vi "test_SomeSessionsRegistered_CallCreateSessionsAndCloseSessionsWithInitializeAndDetach_InitializeAndCloseCalledWithProperBehavior.vi"(11 "error in":errorcluster) -> (4 "pass":bool, 6 "result":string, 15 "error out":errorcluster)   [LabVIEW 2020, in "MeasurementServerTests.lvlib"]
uses:
  MeasurementServerTests.lvlib
  Runtime/MeasurementLink Session Management/Session Reservation/Initialize and Close Session Behavior.ctl
  Runtime/MeasurementLink Session Management/Session Reservation/Session Reservation.lvclass
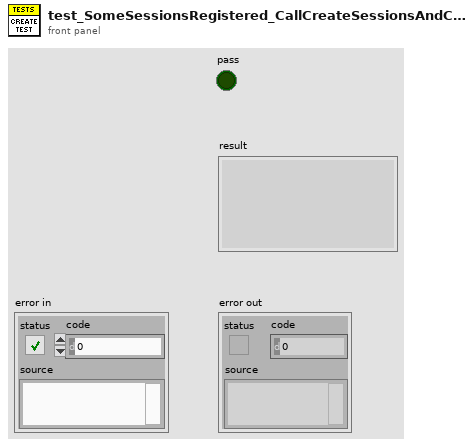
[diagram p1: front panel]
types:
  T1 = typedef "MeasurementLink Session Management.lvlib/Session Reservation.lvclass/Initialize and Close Session Behavior.ctl" = enum16{"Auto", "Initialize and Close", "Attach and Detach", "Initialize and Detach", "Attach and Close"}
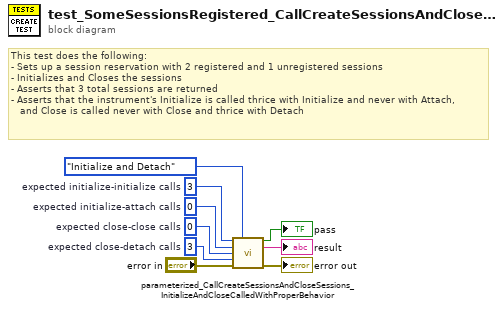
[diagram p0: block diagram]
diagram:
  w5 = u32 3  # expected close-detach calls
  w6 = u32 0  # expected close-close calls
  w7 = u32 0  # expected initialize-attach calls
  w8 = u32 3  # expected initialize-initialize calls
  # "This test does the following:\n- Sets up a session reservation with 2 registered and 1 unregistered sessions\n- Initializes and Closes the sessions\n- Asserts that 3 total sessions are returned\n- Asserts that the instrument's Initialize is called thrice with Initialize and never with Attach,\n   and Close is called never with Close and thrice with Detach"
  n1 = call "parameterized_CallCreateSessionsAndCloseSessions_InitializeAndCloseCalledWithProperBehavior.vi"("expected initialize-initialize calls"=w8, "initialize and close session behavior"=Initialize_and_Close_Session_Behavior."Initialize and Detach", "expected initialize-attach calls"=w7, "expected close-close calls"=w6, "expected close-detach calls"=w5, "error in"="error in") -> ("pass"=→"pass":bool, "result"=→"result":string, "error out"=→"error out":errorcluster)  [unwired: 7 in]
